vi "Reload Config.vi"(8 "error in (no error)":errorcluster, 9 "Promise":refnum<class "Promise.lvclass">, 10 "Config Type":string, 11 "DataProcessor in":refnum<class "DataProcessor.lvclass">) -> (0 "error out":errorcluster, 3 "DataProcessor out":refnum<class "DataProcessor.lvclass">)   [LabVIEW 2020, in "VolatusData.lvlib" / "DataProcessor.lvclass"]
uses:
  DataProcessor.lvclass
  DataProcessor.lvclass/DataProcessor.ctl
  lv-promises/Promises/Error Result/Error Result.lvclass
  lv-promises/Promises/Promise/Promise.lvclass
  C:/dev/lv20CE/relink/lv-promises/Promises/Value/Value.lvclass
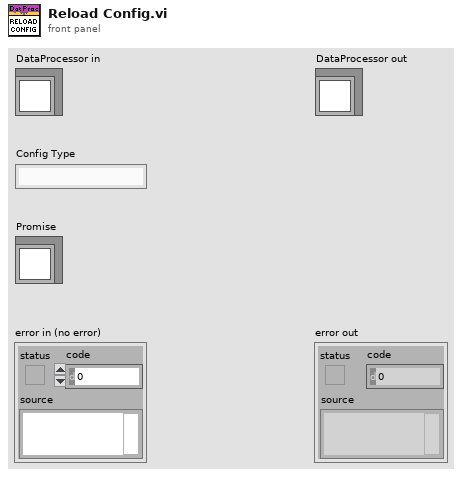
[diagram p1: front panel]
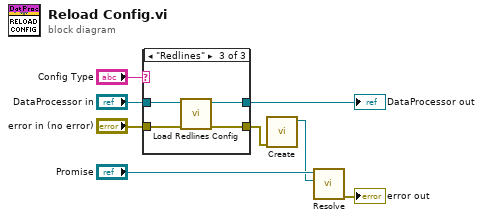
[diagram p0: block diagram]
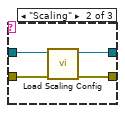
[diagram p3: hidden frame]
diagram:
  n1 = case shown="\"Redlines\"" "Config Type" {
    tunnel: "DataProcessor in" -> [w9 w14 w16]
    tunnel: "error in (no error)" -> [w10 w13 w18]
    tunnel: [w9 w12 w15] -> w5
    tunnel: [w10 w11 w17] -> w3
    frame Default {
    }
    frame "Scaling" {
      n2 = call "Load Scaling Config.vi"("error in (no error)"=w13, "DataProcessor in"=w14) -> ("error out"=w11:errorcluster, "DataProcessor out"=w12:refnum<class "DataProcessor.lvclass">)  [unwired: 8 in]
    }
    frame "Redlines" {
      n3 = call "Load Redlines Config.vi"("error in (no error)"=w18, "DataProcessor in"=w16) -> ("error out"=w17:errorcluster, "DataProcessor out"=w15:refnum<class "DataProcessor.lvclass">)  [unwired: 8 in]
    }
  }
  "DataProcessor out" <- w5
  n4 = call "Create.vi"("error in (no error)"=w3) -> ("Error Result out"=w2:refnum<class "Error Result.lvclass">)  [unwired: 9 in, 1 out]
  n5 = call "Resolve.vi"("Result"=w2, "Promise in"="Promise") -> ("error out"=→"error out":errorcluster)  [unwired: 8 in, 1 out]
